vi "Read.vi"(6 "timeout (ms)":i32=5000, 8 "error in (no error)":errorcluster, 10 "number of samples":i32=10000, 11 "9770 API in":refnum<class "9770 API.lvclass">) -> (0 "error out":errorcluster, 1 "PeakRFPower":dbl, 2 "Waveform":waveform(cdb), 3 "9770 API out":refnum<class "9770 API.lvclass">, 4 "samples remaining":u32, 5 "ChannelName":string)   [LabVIEW 2017, in "9770 API.lvclass"]
uses:
  <vilib>/addons/InsightCM/Devices/Shared/Emsa/Emsa9770API/9770 API.lvclass
  <vilib>/addons/InsightCM/Devices/Shared/Emsa/Emsa9770API/9770 API.lvclass/9770 API.ctl
  <vilib>/Utility/error.llb/Error Cluster From Error Code.vi
  <vilib>/rvi/errors/niLvFpgaAdjustHostInterfaceError.vi
  <vilib>/rvi/interface/nirviMethod/nirviMethod.xnode
  <vilib>/addons/InsightCM/Devices/Shared/Emsa/Emsa9770API/controls/FPGATypeDef.ctl
  <vilib>/rvi/interface/nirviReadWriteControl/nirviReadWriteControl.xnode
  NiFpgaLv.dll
  <vilib>/rvi/interface/Simulation/niFpgaSimulationCallBeginRW.vi
  <vilib>/FPGAPlugInAG/Dynamic/niLvFpga_ReadFifo_Dynamic.vi
  <vilib>/rvi/errors/niLvFpgaMergeErrorWithErrorCode.vi
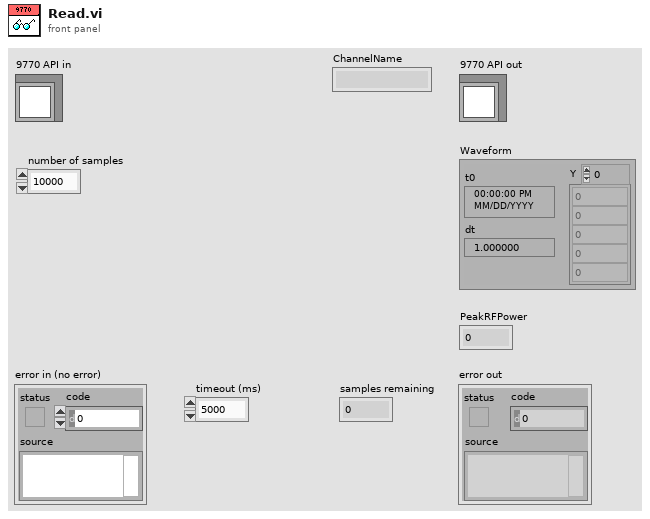
[diagram p1: front panel]
types:
  T1 = typedef "9770 API.lvclass/FPGATypeDef.ctl" = refnum<k20>
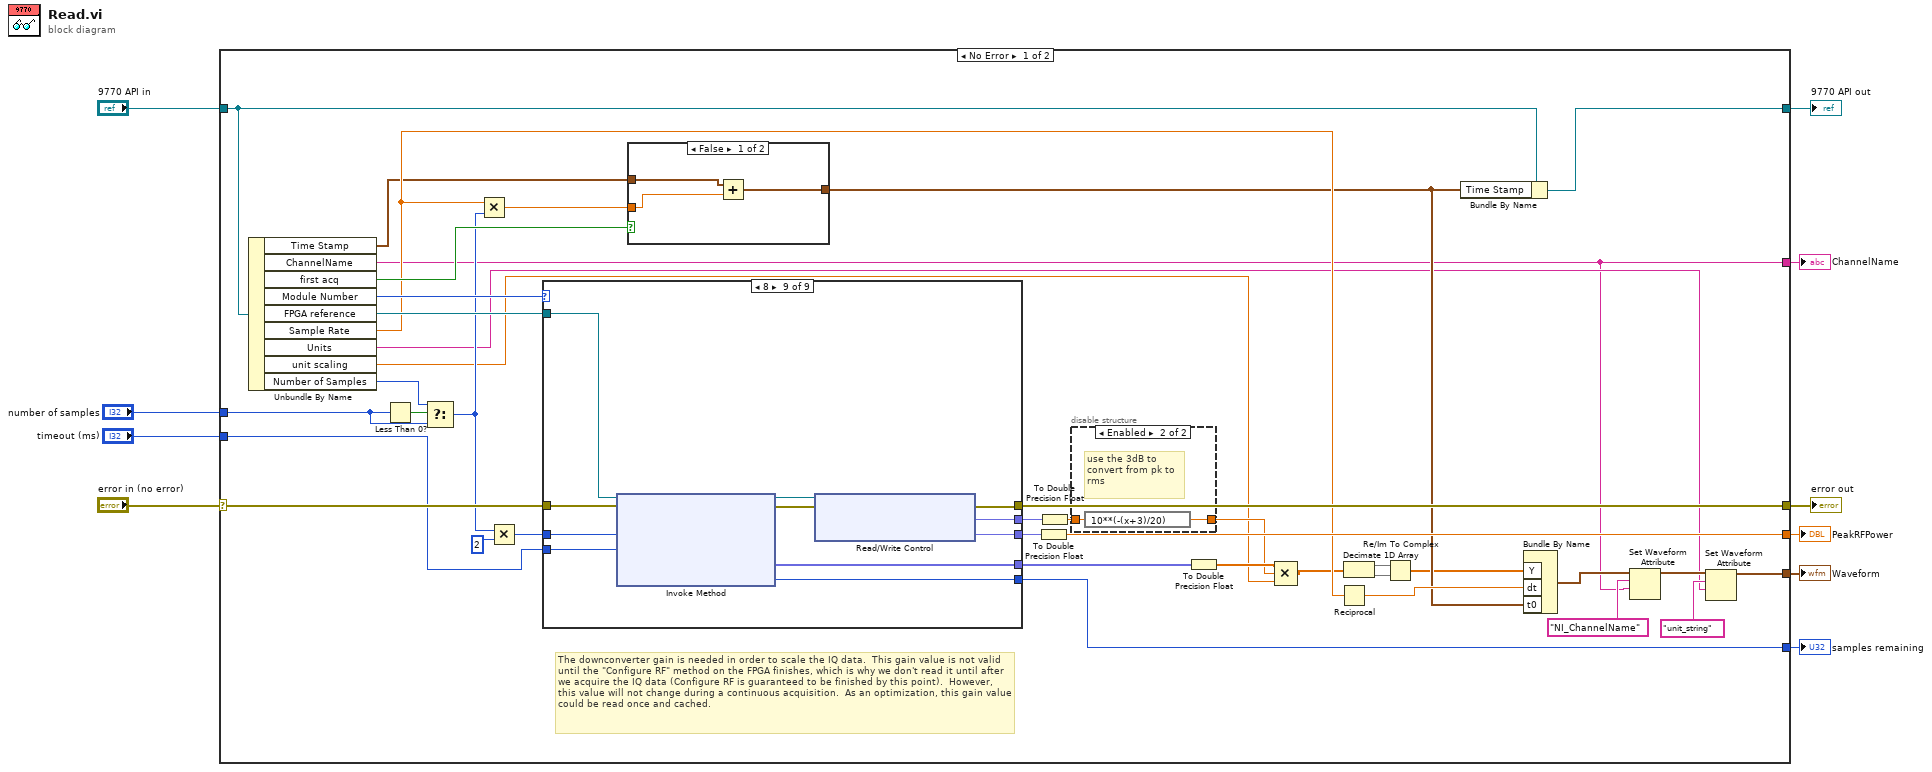
[diagram p0: block diagram]
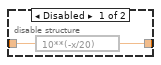
[diagram p2: hidden frame]
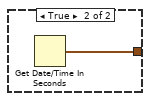
[diagram p3: hidden frame]
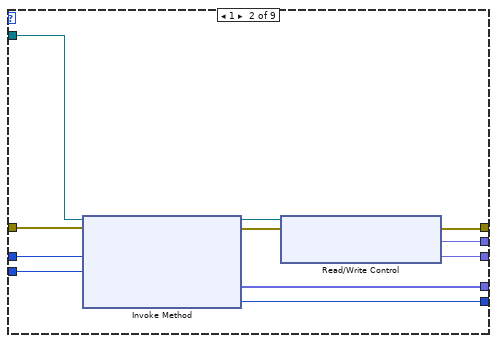
[diagram p5: hidden frame]
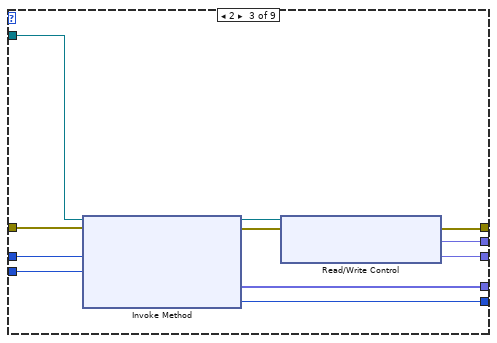
[diagram p6: hidden frame]
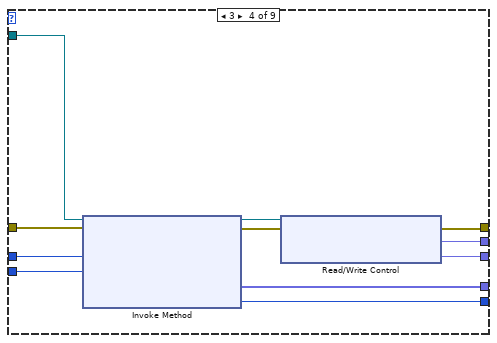
[diagram p7: hidden frame]
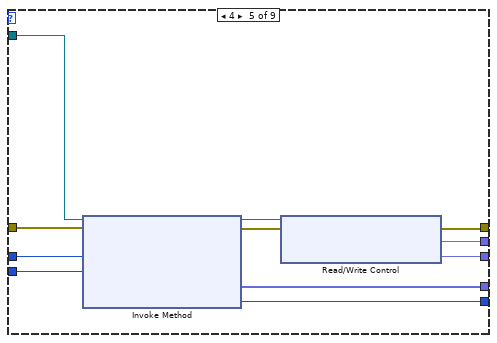
[diagram p8: hidden frame]
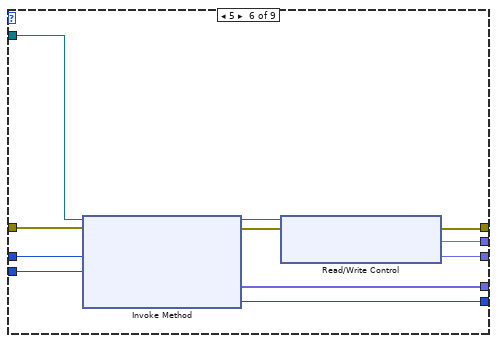
[diagram p9: hidden frame]
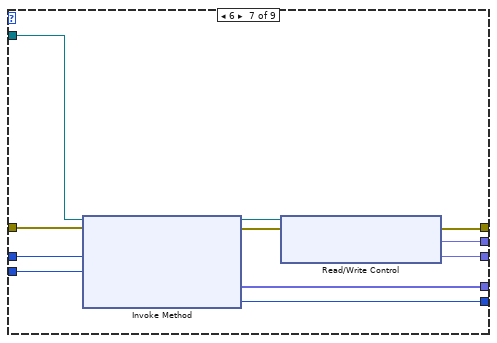
[diagram p10: hidden frame]
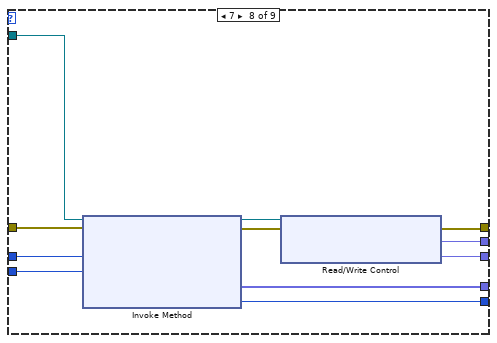
[diagram p11: hidden frame]
diagram:
  n1 = case shown="No Error" "error in (no error)" {
    selector: "error in (no error)" -> [w47 w148]
    tunnel: [w46 w148] -> w9
    tunnel: [w25 w147] -> w7
    tunnel: "9770 API in" -> [w27 w147]
    tunnel: "number of samples" -> [w33 _]
    tunnel: "timeout (ms)" -> [w43 _]
    tunnel: [w36 _] -> w4
    tunnel: [w18 _] -> w3
    tunnel: [w24 _] -> w2
    tunnel: [w11 _] -> w1
    frame No Error {
      # "The downconverter gain is needed in order to scale the IQ data.  This gain value is not valid until the \"Configure RF\" method on the FPGA finishes, which is why we don't read it until after we acquire the IQ data (Configure RF is guaranteed to be finished by this point).  However, this value will not change during a continuous acquisition.  As an optimization, this gain value could be read once and cached."
      n2 = Unbundle By Name(w27) -> ("Time Stamp"=w28:timestamp, "ChannelName"=w11:string, "first acq"=w32:bool, "Module Number"=w49:u32, "FPGA reference"=w48:T1, "Sample Rate"=w30:dbl, "Units"=w16:string, "unit scaling"=w12:dbl, "Number of Samples"=w34:i32)
      n3 = Less Than 0?(x=w33) -> (x < 0?=w35:bool)
      n4 = Select(t=w34, s=w35, f=w33) -> (s? t:f=w31:i32)
      n5 = Multiply(x=w30, y=w31) -> (x*y=w29:dbl)
      n6 = Multiply(x=w31, y=2) -> (x*y=w44:i32)
      n7 = case shown="8" w49 {
        tunnel: w48 -> [_ w65 w76 w87 w98 w109 w120 w131 w142]
        tunnel: w47 -> [w58 w67 w78 w89 w100 w111 w122 w133 w144]
        tunnel: [w58 w66 w77 w88 w99 w110 w121 w132 w143] -> w46
        tunnel: w44 -> [_ w64 w75 w86 w97 w108 w119 w130 w141]
        tunnel: w43 -> [_ w63 w74 w85 w96 w107 w118 w129 w140]
        tunnel: [_ w62 w73 w84 w95 w106 w117 w128 w139] -> w38
        tunnel: [_ w61 w72 w83 w94 w105 w116 w127 w138] -> w37
        tunnel: [_ w60 w71 w82 w93 w104 w115 w126 w137] -> w41
        tunnel: [_ w59 w70 w81 w92 w103 w114 w125 w136] -> w24
        frame 0, Default {
        }
        frame 1 {
          n8 = xnode "Invoke Method"("FPGA VI Reference In"=w65, "error in"=w67, "Number of Elements"=w64, "Timeout (ms)"=w63) -> ("FPGA VI Reference Out"=w68:T1, "error out"=w69:errorcluster, "Data"=w60:fxp<+/-,20,1>[], "Elements Remaining"=w59:u32)
          n9 = xnode "Read/Write Control"("FPGA VI Reference In"=w68, "error in"=w69) -> ("error out"=w66:errorcluster, "Downconverter Gain (dB) 1"=w62:fxp<+/-,15,8>, "PeakRFPower 1"=w61:fxp<+/-,12,8>)  [unwired: 1 out]
        }
        frame 2 {
          n10 = xnode "Invoke Method"("FPGA VI Reference In"=w76, "error in"=w78, "Number of Elements"=w75, "Timeout (ms)"=w74) -> ("FPGA VI Reference Out"=w79:T1, "error out"=w80:errorcluster, "Data"=w71:fxp<+/-,20,1>[], "Elements Remaining"=w70:u32)
          n11 = xnode "Read/Write Control"("FPGA VI Reference In"=w79, "error in"=w80) -> ("error out"=w77:errorcluster, "Downconverter Gain (dB) 2"=w73:fxp<+/-,15,8>, "PeakRFPower 2"=w72:fxp<+/-,12,8>)  [unwired: 1 out]
        }
        frame 3 {
          n12 = xnode "Invoke Method"("FPGA VI Reference In"=w87, "error in"=w89, "Number of Elements"=w86, "Timeout (ms)"=w85) -> ("FPGA VI Reference Out"=w90:T1, "error out"=w91:errorcluster, "Data"=w82:fxp<+/-,20,1>[], "Elements Remaining"=w81:u32)
          n13 = xnode "Read/Write Control"("FPGA VI Reference In"=w90, "error in"=w91) -> ("error out"=w88:errorcluster, "Downconverter Gain (dB) 3"=w84:fxp<+/-,15,8>, "PeakRFPower 3"=w83:fxp<+/-,12,8>)  [unwired: 1 out]
        }
        frame 4 {
          n14 = xnode "Invoke Method"("FPGA VI Reference In"=w98, "error in"=w100, "Number of Elements"=w97, "Timeout (ms)"=w96) -> ("FPGA VI Reference Out"=w101:T1, "error out"=w102:errorcluster, "Data"=w93:fxp<+/-,20,1>[], "Elements Remaining"=w92:u32)
          n15 = xnode "Read/Write Control"("FPGA VI Reference In"=w101, "error in"=w102) -> ("error out"=w99:errorcluster, "Downconverter Gain (dB) 4"=w95:fxp<+/-,15,8>, "PeakRFPower 4"=w94:fxp<+/-,12,8>)  [unwired: 1 out]
        }
        frame 5 {
          n16 = xnode "Invoke Method"("FPGA VI Reference In"=w109, "error in"=w111, "Number of Elements"=w108, "Timeout (ms)"=w107) -> ("FPGA VI Reference Out"=w112:T1, "error out"=w113:errorcluster, "Data"=w104:fxp<+/-,20,1>[], "Elements Remaining"=w103:u32)
          n17 = xnode "Read/Write Control"("FPGA VI Reference In"=w112, "error in"=w113) -> ("error out"=w110:errorcluster, "Downconverter Gain (dB) 5"=w106:fxp<+/-,15,8>, "PeakRFPower 5"=w105:fxp<+/-,12,8>)  [unwired: 1 out]
        }
        frame 6 {
          n18 = xnode "Invoke Method"("FPGA VI Reference In"=w120, "error in"=w122, "Number of Elements"=w119, "Timeout (ms)"=w118) -> ("FPGA VI Reference Out"=w123:T1, "error out"=w124:errorcluster, "Data"=w115:fxp<+/-,20,1>[], "Elements Remaining"=w114:u32)
          n19 = xnode "Read/Write Control"("FPGA VI Reference In"=w123, "error in"=w124) -> ("error out"=w121:errorcluster, "Downconverter Gain (dB) 6"=w117:fxp<+/-,15,8>, "PeakRFPower 6"=w116:fxp<+/-,12,8>)  [unwired: 1 out]
        }
        frame 7 {
          n20 = xnode "Invoke Method"("FPGA VI Reference In"=w131, "error in"=w133, "Number of Elements"=w130, "Timeout (ms)"=w129) -> ("FPGA VI Reference Out"=w134:T1, "error out"=w135:errorcluster, "Data"=w126:fxp<+/-,20,1>[], "Elements Remaining"=w125:u32)
          n21 = xnode "Read/Write Control"("FPGA VI Reference In"=w134, "error in"=w135) -> ("error out"=w132:errorcluster, "Downconverter Gain (dB) 7"=w128:fxp<+/-,15,8>, "PeakRFPower 7"=w127:fxp<+/-,12,8>)  [unwired: 1 out]
        }
        frame 8 {
          n22 = xnode "Invoke Method"("FPGA VI Reference In"=w142, "error in"=w144, "Number of Elements"=w141, "Timeout (ms)"=w140) -> ("FPGA VI Reference Out"=w145:T1, "error out"=w146:errorcluster, "Data"=w137:fxp<+/-,20,1>[], "Elements Remaining"=w136:u32)
          n23 = xnode "Read/Write Control"("FPGA VI Reference In"=w145, "error in"=w146) -> ("error out"=w143:errorcluster, "Downconverter Gain (dB) 8"=w139:fxp<+/-,15,8>, "PeakRFPower 8"=w138:fxp<+/-,12,8>)  [unwired: 1 out]
        }
      }
      n24 = case shown="False" w32 {
        tunnel: [w55 w57] -> w26
        tunnel: w28 -> [w56 _]
        tunnel: w29 -> [w54 _]
        frame False {
          n25 = Add(x=w56, y=w54) -> (x+y=w55:timestamp)
        }
        frame True {
          n26 = Get Date/Time In Seconds() -> (seconds since 1Jan1904=w57:timestamp)
        }
      }
      n27 = To Double Precision Float(number=w37) -> (double precision float=w36:dbl)
      n28 = To Double Precision Float(number=w38) -> (double precision float=w42:dbl)
      n29 = disable-structure shown="Enabled" {
        disable-tunnel: w42 -> [w51 w53]
        disable-tunnel: [w50 w52] -> w14
        frame Disabled {
          n30 = expression code="10**(-x/20)"(w51) -> (w50:dbl)
        }
        frame Enabled {
          # "use the 3dB to convert from pk to rms"
          n31 = expression code="10**(-(x+3)/20)"(w53) -> (w52:dbl)
        }
      }
      n32 = To Double Precision Float(number=w41) -> (double precision float=w15:dbl[])
      n33 = Compound Arithmetic op=MULTIPLY(w15, w14, w12) -> (w13:dbl[])
      n34 = Reciprocal(x=w30) -> (1/x=w40:dbl)
      n35 = Decimate 1D Array(w13) -> (w23:dbl[], w39:dbl[])
      n36 = Re/Im To Complex(1:w39, 2:w23) -> (0:w22:cdb[])
      n37 = Bundle By Name(cluster=w27, "Time Stamp"=w26) -> (w25:refnum<class "9770 API.lvclass">)
      n38 = Bundle By Name("Y"=w22, "dt"=w40, "t0"=w26) -> (w21:waveform(cdb))  [unwired: 1 in]
      n39 = Set Waveform Attribute(5:w11, 6:"NI_ChannelName" ("name"), 7:w21) -> (3:w19:waveform(cdb))  [unwired: 1 in, 2 out]
      n40 = Set Waveform Attribute(5:w16, 6:"unit_string" ("name"), 7:w19) -> (3:w18:waveform(cdb))  [unwired: 1 in, 2 out]
    }
    frame Error {
    }
  }
  "error out" <- w9
  "9770 API out" <- w7
  "PeakRFPower" <- w4
  "Waveform" <- w3
  "samples remaining" <- w2
  "ChannelName" <- w1
